vi "Global_System_Checks.vi"() -> ()   [LabVIEW 2017]
uses:
  Control 1.ctl
panel:
  out "System Enabled":T1
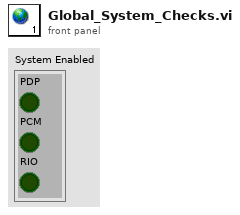
[diagram p1: front panel]
types:
  T1 = typedef "Control 1.ctl" = cluster{"PDP ":bool, "PCM":bool, "RIO":bool}
diagram:
